vi "Get Icon Size.vi"(8 "error in (no error)":errorcluster, 11 "Control in":refnum<class "Control.lvclass">) -> (0 "error out":errorcluster, 2 "Icon Size":cluster{"Width":i32, "Height":i32} caption="Size", 3 "Control out":refnum<class "Control.lvclass">)   [LabVIEW 2012, in "Control.lvclass"]
doc: "Gets the icon size."
uses:
  Control.lvclass
  Control.lvclass/Control.ctl
  <userlib>/BitMan/BitMap class/BitMap.lvclass
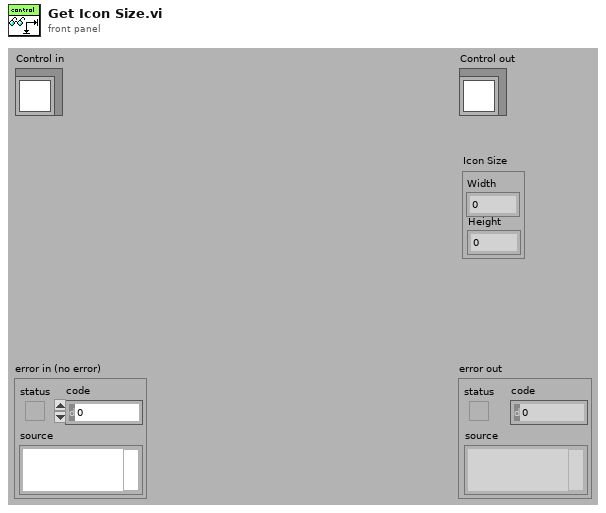
[diagram p1: front panel]
types:
  T1 = typedef "BitMan Lib.lvlib/Size type.ctl" = cluster{"Width":i32, "Height":i32}
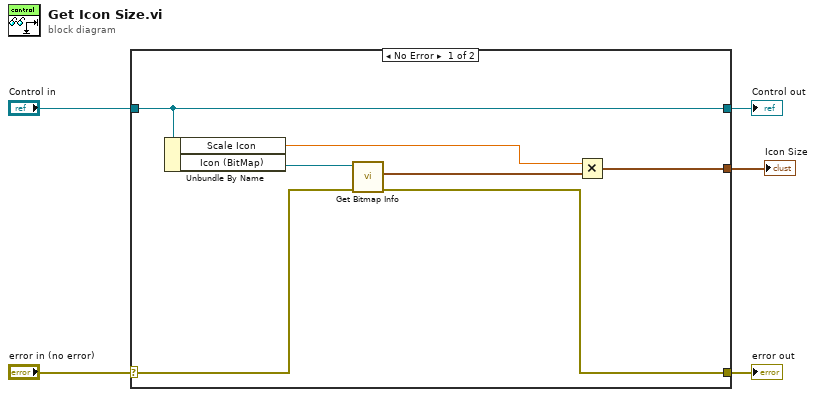
[diagram p0: block diagram]
diagram:
  n1 = case shown="No Error" "error in (no error)" {
    selector: "error in (no error)" -> [w7 w14]
    tunnel: [w6 w14] -> w4
    tunnel: [w8 w13] -> w2
    tunnel: "Control in" -> [w8 w13]
    tunnel: [w10 _] -> w1
    frame No Error {
      n2 = Unbundle By Name(w8) -> ("Scale Icon"=w9:dbl, "Icon (BitMap)"=w12:refnum<class "BitMap.lvclass">)
      n3 = call <userlib>:"Get Bitmap Info.vi"("error in (no error)"=w7, "BitMap in"=w12) -> ("error out"=w6:errorcluster, "Size"=w11:T1)  [unwired: 8 out]
      n4 = Multiply(x=w9, y=w11) -> (x*y=w10:cluster{"Width":dbl, "Height":dbl})
    }
    frame Error {
    }
  }
  "error out" <- w4
  "Control out" <- w2
  "Icon Size" <- w1
